vi "sv_UFF58 Set Channel Length.vi"(0 "channel refnum":refnum<k20>, 5 "channel length":i32, 11 "error in":errorcluster caption="error in (no error)") -> (4 "channel refnum":refnum<k20>, 15 "error out":errorcluster)   [LabVIEW 2017, in "SoundVib_UFF58.lvlib"]
doc: "This VI returns the <B>channel length</B> for the given <B>channel refnum</B>"
uses:
  <vilib>/addons/Sound and Vibration/svt_UFF58/SoundVib_UFF58.lvlib
  <vilib>/Platform/storage/Storage.llb/Set Property (I32).vi
  <vilib>/Platform/storage/Storage.llb/Get Property (Storage Refnum).vi
  <vilib>/Platform/storage/Storage.llb/Get Property (Storage Refnums).vi
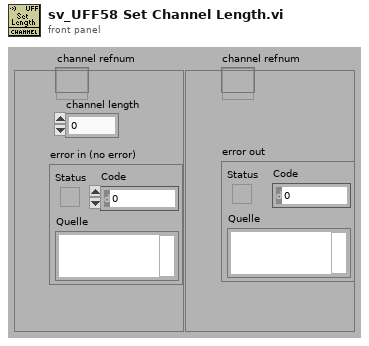
[diagram p1: front panel]
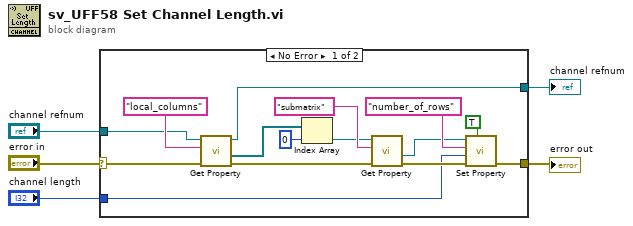
[diagram p0: block diagram]
diagram:
  n1 = case shown="No Error" "error in" {
    selector: "error in" -> [w12 w22]
    tunnel: [w11 w22] -> w5
    tunnel: "channel refnum" -> [w14 w21]
    tunnel: [w13 w21] -> w3
    tunnel: "channel length" -> [w7 _]
    frame No Error {
      n2 = call-poly <vilib>:"Get Property.vi"("error in (no error)"=w12, "Property name"="local_columns" ("property name"), "storage refnum"=w14) -> ("error out"=w20:errorcluster, "Value"=w16:refnum<k20>[], "storage refnum out"=w13:refnum<k20>)  [unwired: 6 in]
      n3 = Index Array(array=w16, index=0 ("Index")) -> (element=w18:refnum<k20>)
      n4 = call-poly <vilib>:"Get Property.vi"("error in (no error)"=w20, "Property name"="submatrix" ("property name"), "storage refnum"=w18) -> ("error out"=w10:errorcluster, "Value"=w8:refnum<k20>)  [unwired: 6 in, 1 out]
      n5 = call-poly <vilib>:"Set Property.vi"("Create if not found (no:F)"=TRUE, "error in (no error)"=w10, "Value"=w7, "Property name"="number_of_rows" ("property name"), "storage refnum"=w8) -> ("error out"=w11:errorcluster)  [unwired: 5 in, 1 out]
    }
    frame Error {
    }
  }
  "error out" <- w5
  "channel refnum" <- w3
